vi "Configure Measurement.vi"   [LabVIEW 2015, in "Template - Counter.lvlib"]
doc: "Choose to configure any type of measurement the instrument is capable of making."
uses:
  <instrlib>/_Template - Counter/Template - Counter.lvlib
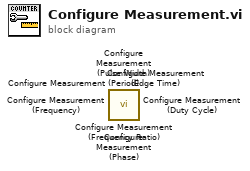
[diagram p0: block diagram]
diagram:
  n1 = call <instrlib>:"Configure Measurement (Frequency Ratio).vi"() -> ()  [unwired: 10 in, 2 out]
  n2 = call <instrlib>:"Configure Measurement (Edge Time).vi"() -> ()  [unwired: 10 in, 2 out]
  n3 = call <instrlib>:"Configure Measurement (Frequency).vi"() -> ()  [unwired: 10 in, 2 out]
  n4 = call <instrlib>:"Configure Measurement (Duty Cycle).vi"() -> ()  [unwired: 10 in, 2 out]
  n5 = call <instrlib>:"Configure Measurement (Period).vi"() -> ()  [unwired: 10 in, 2 out]
  n6 = call <instrlib>:"Configure Measurement (Pulse Width).vi"() -> ()  [unwired: 10 in, 2 out]
  n7 = call <instrlib>:"Configure Measurement (Phase).vi"() -> ()  [unwired: 10 in, 2 out]
